vi "Ball_Create.vi"(0 "reference in":refnum<class "Ball.lvclass">, 5 "error in (no error)":errorcluster) -> (14 "reference out":refnum<class "Ball.lvclass">, 19 "error out":errorcluster)   [LabVIEW 2018, in "Ball.lvclass"]
uses:
  Ball.lvclass
  Object_class/Object.lvclass
  C:/Users/Ronaldo/Desktop/SSL_AI/SSL_AI-dev/Object_class/Object.lvclass
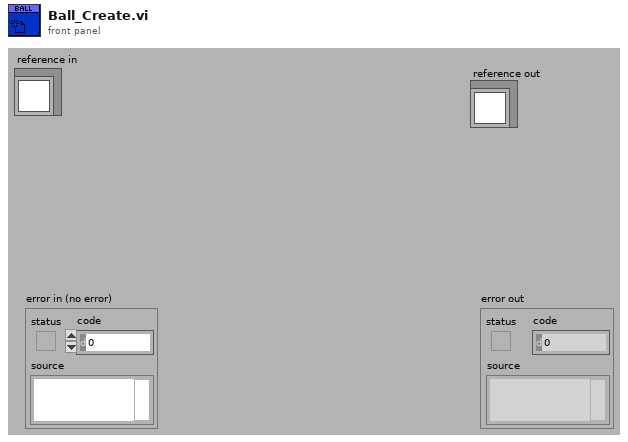
[diagram p1: front panel]
types:
  T1 = typedef "Ball.lvclass/ObjectAttributes.ctl" = cluster{"Base class":T2}
  T2 = typedef "Object.lvclass/ObjectAttributes.ctl" = cluster{"None":bool}
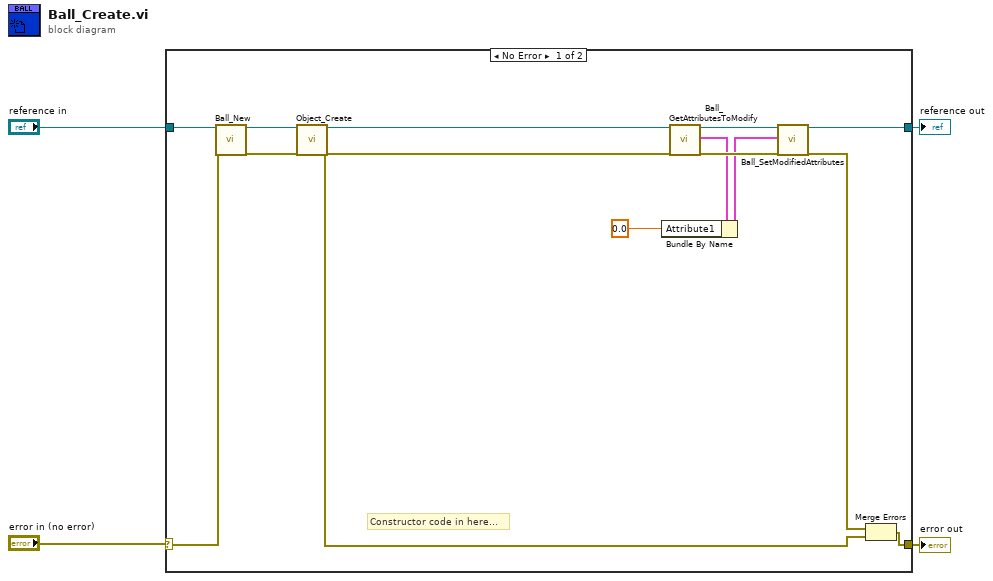
[diagram p0: block diagram]
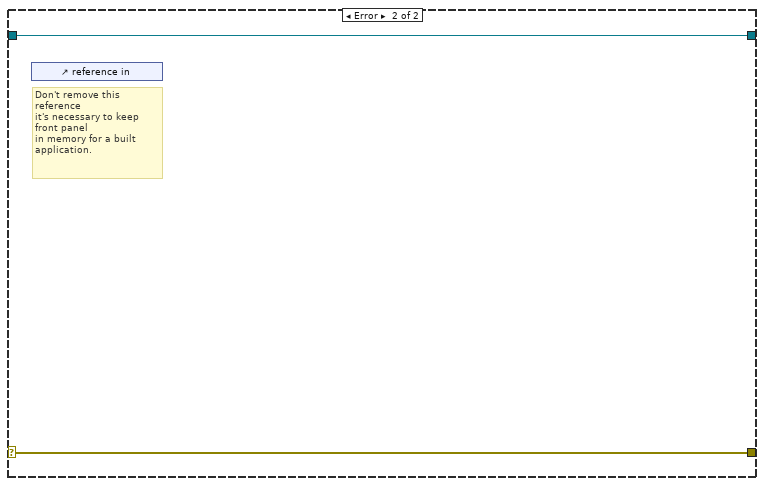
[diagram p2: hidden frame]
diagram:
  n1 = case shown="No Error" "error in (no error)" {
    selector: "error in (no error)" -> [w16 w20]
    tunnel: [w9 w20] -> w3
    tunnel: [w14 w19] -> w2
    tunnel: "reference in" -> [w6 w19]
    frame No Error {
      # "Constructor code in here..."
      n2 = call "Ball_New.vi"("reference in"=w6, "error in (no error)"=w16) -> ("reference out"=w11:refnum<class "Ball.lvclass">, "error out"=w15:errorcluster)  [unwired: 14 in, 2 out]
      n3 = call "Object_Create.vi"("reference in"=w11, "error in (no error)"=w15) -> ("reference out"=w10:refnum<class "Ball.lvclass">, "error out"=w7:errorcluster)  [unwired: 16 in]
      n4 = call "Ball_GetAttributesToModify.vi"("reference in"=w10, "error in (no error)"=w7) -> ("reference out"=w18:refnum<class "Ball.lvclass">, "Attributes"=w13:T1, "error out"=w17:errorcluster)  [unwired: 14 in, 1 out]
      n5 = Bundle By Name(cluster=w13, "Attribute1"=0.0 ("Base class.Attribute1")) -> (w12:T1)
      n6 = call "Ball_SetModifiedAttributes.vi"("reference in"=w18, "Attributes"=w12, "error in (no error)"=w17) -> ("reference out"=w14:refnum<class "Ball.lvclass">, "error out"=w8:errorcluster)  [unwired: 15 in]
      n7 = Merge Errors(w8, w7) -> (w9:errorcluster)
    }
    frame Error {
      # "Don't remove this reference\nit's necessary to keep front panel\nin memory for a built application."
      n8 = control-ref of="reference in"() -> ()  [unwired: 1 out]
    }
  }
  "error out" <- w3
  "reference out" <- w2
